vi "oax_Load Data (Analog Tacho, Single channel).vi"(0 "Data Path In":path, 11 "error in (no error)":errorcluster) -> (3 "channel name":string[](array[string]), 4 "waveform signal":waveform(dbl), 8 "analog tacho signal":waveform(dbl), 14 "tacho info":T1 {"slope (Rising)" items=["Rising", "Falling"]}, 15 "error out":errorcluster)   [LabVIEW 2017]
doc: "Specify the .dat file to load vibration and tachometer data from."
uses:
  <vilib>/addons/Sound and Vibration/svt_Calibration/SVL Scale Voltage to EU (1 Ch).vi
  <vilib>/addons/_NISVFA/_Shared subVIs/Common/svc_Set SV Channel Info.vi
  <vilib>/addons/_NISVFA/_Shared subVIs/Common/svc_Set SV Channel Info (variant).vi
  <vilib>/addons/_NISVFA/_Shared subVIs/Common/SVL Set dB Reference (variant).vi
  <vilib>/addons/_NISVFA/_Shared subVIs/Common/svc_Caller VI Returned in Error Source.vi
  <vilib>/addons/_NISVFA/_Shared subVIs/Common/svc_Engineering Units to Unit Label.vi
  <vilib>/addons/_NISVFA/_Shared subVIs/Common/svc_Set dB ref if Pascal.vi
  <vilib>/addons/_NISVFA/_Shared subVIs/Common/svc_Compute Scale Factor to Convert C to EU.vi
  <vilib>/addons/_NISVFA/_Shared subVIs/Common/svc_Compute Scale Factor to Convert V to EU.vi
  <vilib>/addons/Sound and Vibration/svt_Calibration/SoundVib_Calibration.lvlib
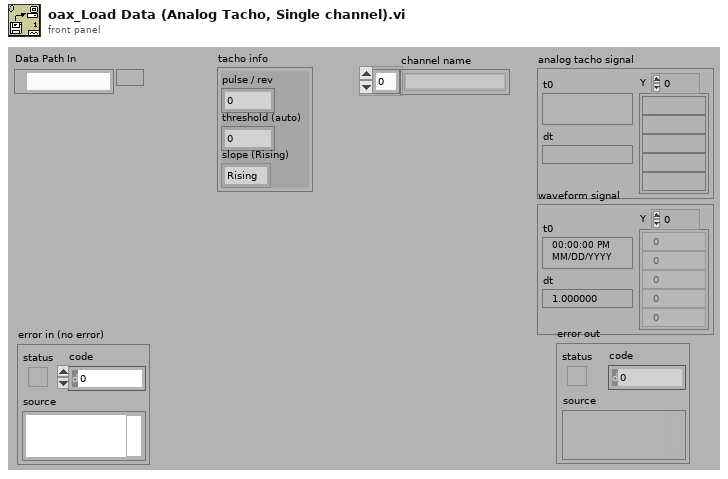
[diagram p1: front panel]
types:
  T1 = cluster{"pulse / rev":i32, "threshold (auto)":dbl, "slope (Rising)":u16}
  T2 = enum16{"open", "open or create", "create or replace", "create", "open (read only)"}
  T3 = typedef "svc_Channel Info.ctl" = cluster{"sensor sensitivity":dbl, "engineering units":T4, "dB reference":dbl, "custom label":string, "weighting filter":T5, "pregain":dbl}
  T4 = typedef "svc_Engineering Units Text Ring.ctl" = u16
  T5 = typedef "svc_Weighting Filter Text Ring.ctl" = u16
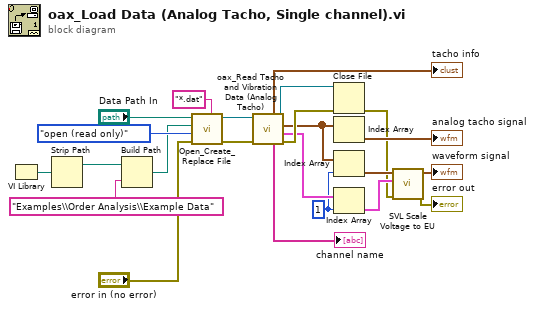
[diagram p0: block diagram]
diagram:
  w1 = 1 ("index")
  n1 = VI Library() -> (path=w12:path)
  n2 = Strip Path(path=w12) -> (stripped path=w11:path)  [unwired: 1 out]
  n3 = Build Path(base path=w11, name or relative path="Examples\\Order Analysis\\Example Data") -> (appended path=w9:path)
  n4 = call <vilib>:"Open_Create_Replace File.vi"("pattern"="*.dat", "error in (no error)"="error in (no error)", "function (open:0)"=T2."open (read only)", "start path  (Not A Path)"=w9, "file path"="Data Path In") -> ("error out"=w20:errorcluster, "refnum"=w21:refnum<file>)  [unwired: 3 in, 2 out]
  n5 = call <vilib>:"oax_Read Tacho and Vibration Data (Analog Tacho).vi"("error in (no error)"=w20, "refnum"=w21) -> ("error out"=w13:errorcluster, "channel info"=w6:T3[], "waveform data"=w7:waveform(dbl)[], "refnum out"=w14:refnum<file>, "channel name"=→"channel name":string[], "tacho info"=→"tacho info":T1)  [unwired: 4 in]
  n6 = Close File(refnum=w14, error in=w13) -> (error out=w3:errorcluster)  [unwired: 1 out]
  n7 = Index Array(array=w7) -> (element=→"analog tacho signal":waveform(dbl))  [unwired: 1 in]
  n8 = Index Array(array=w7, index=w1) -> (element=w5:waveform(dbl))
  n9 = Index Array(array=w6, index=w1) -> (element=w4:T3)
  n10 = call-poly <vilib>:"SVL Scale Voltage to EU.vi"("error in (no error)"=w3, "channel info"=w4, "signal [V]"=w5) -> ("error out"=→"error out":errorcluster, "scaled signal [EU]"=→"waveform signal":waveform(dbl))  [unwired: 6 in, 1 out]
